vi "加速度曲線生成.vi"(0 "X Time":T1={"Time 1"=30.0, "Time 2"=60.0, "Time 3"=70.0, "Time 4"=80.0, "Time 5"=120.0, "Time 6"=180.0, "Time 7"=220.0, "Time 8"=300.0} {"Time 8" step=100.0; "Time 7" step=100.0; "Time 6" step=100.0; "Time 5" step=100.0; "Time 4" step=100.0; "Time 3" step=100.0; "Time 2" step=100.0; "Time 1" step=100.0}, 1 "Y Velocity":T2={"Speed 1"=70.0, "Speed 2"=-95.0, "Speed 3"=50.0, "Speed 4"=-50.0, "Speed 5"=60.0, "Speed 6"=-60.0, "Speed 7"=102.0, "Speed 8"=-80.0} {"Speed 8" step=100.0; "Speed 7" step=100.0; "Speed 6" step=100.0; "Speed 5" step=100.0; "Speed 4" step=100.0; "Speed 3" step=100.0; "Speed 2" step=100.0; "Speed 1" step=100.0}) -> (2 "Ideal Move":dbl[](array[numeric]), 3 "Ideal Acc":dbl[](array[numeric]), 4 "Voltage 1":dbl[](array[numeric]), 5 "Voltage 2":dbl[](array[numeric]), 6 "Voltage 3":dbl[](array[numeric]), 7 "Ideal Velocity":dbl[](array[numeric]))   [LabVIEW 2019]
uses:
  <vilib>/Analysis/NI_AALPro.lvlib
panel:
  out "Ideal Move Position Graph":cluster{"Speed":dbl[], "Position":dbl[]}(graph)
  out "Ideal S Graph":cluster{"Speed":dbl[], "Position":dbl[]}(graph)
  out "Ideal Velocity Graph":cluster{"Speed":dbl[], "Position":dbl[]}(graph)
  out "Ideal Axis 3 Voltage Position":cluster{dbl[], dbl[]}(graph)
  out "Ideal Axis 2 Voltage Position":cluster{dbl[], dbl[]}(graph)
  out "Ideal  Axis 1 Voltage Position":cluster{dbl[], dbl[]}(graph)
  out "Ideal Acceleration Graph":cluster{"Speed":dbl[], "Position":dbl[]}(graph)
  # "1mm/sec"
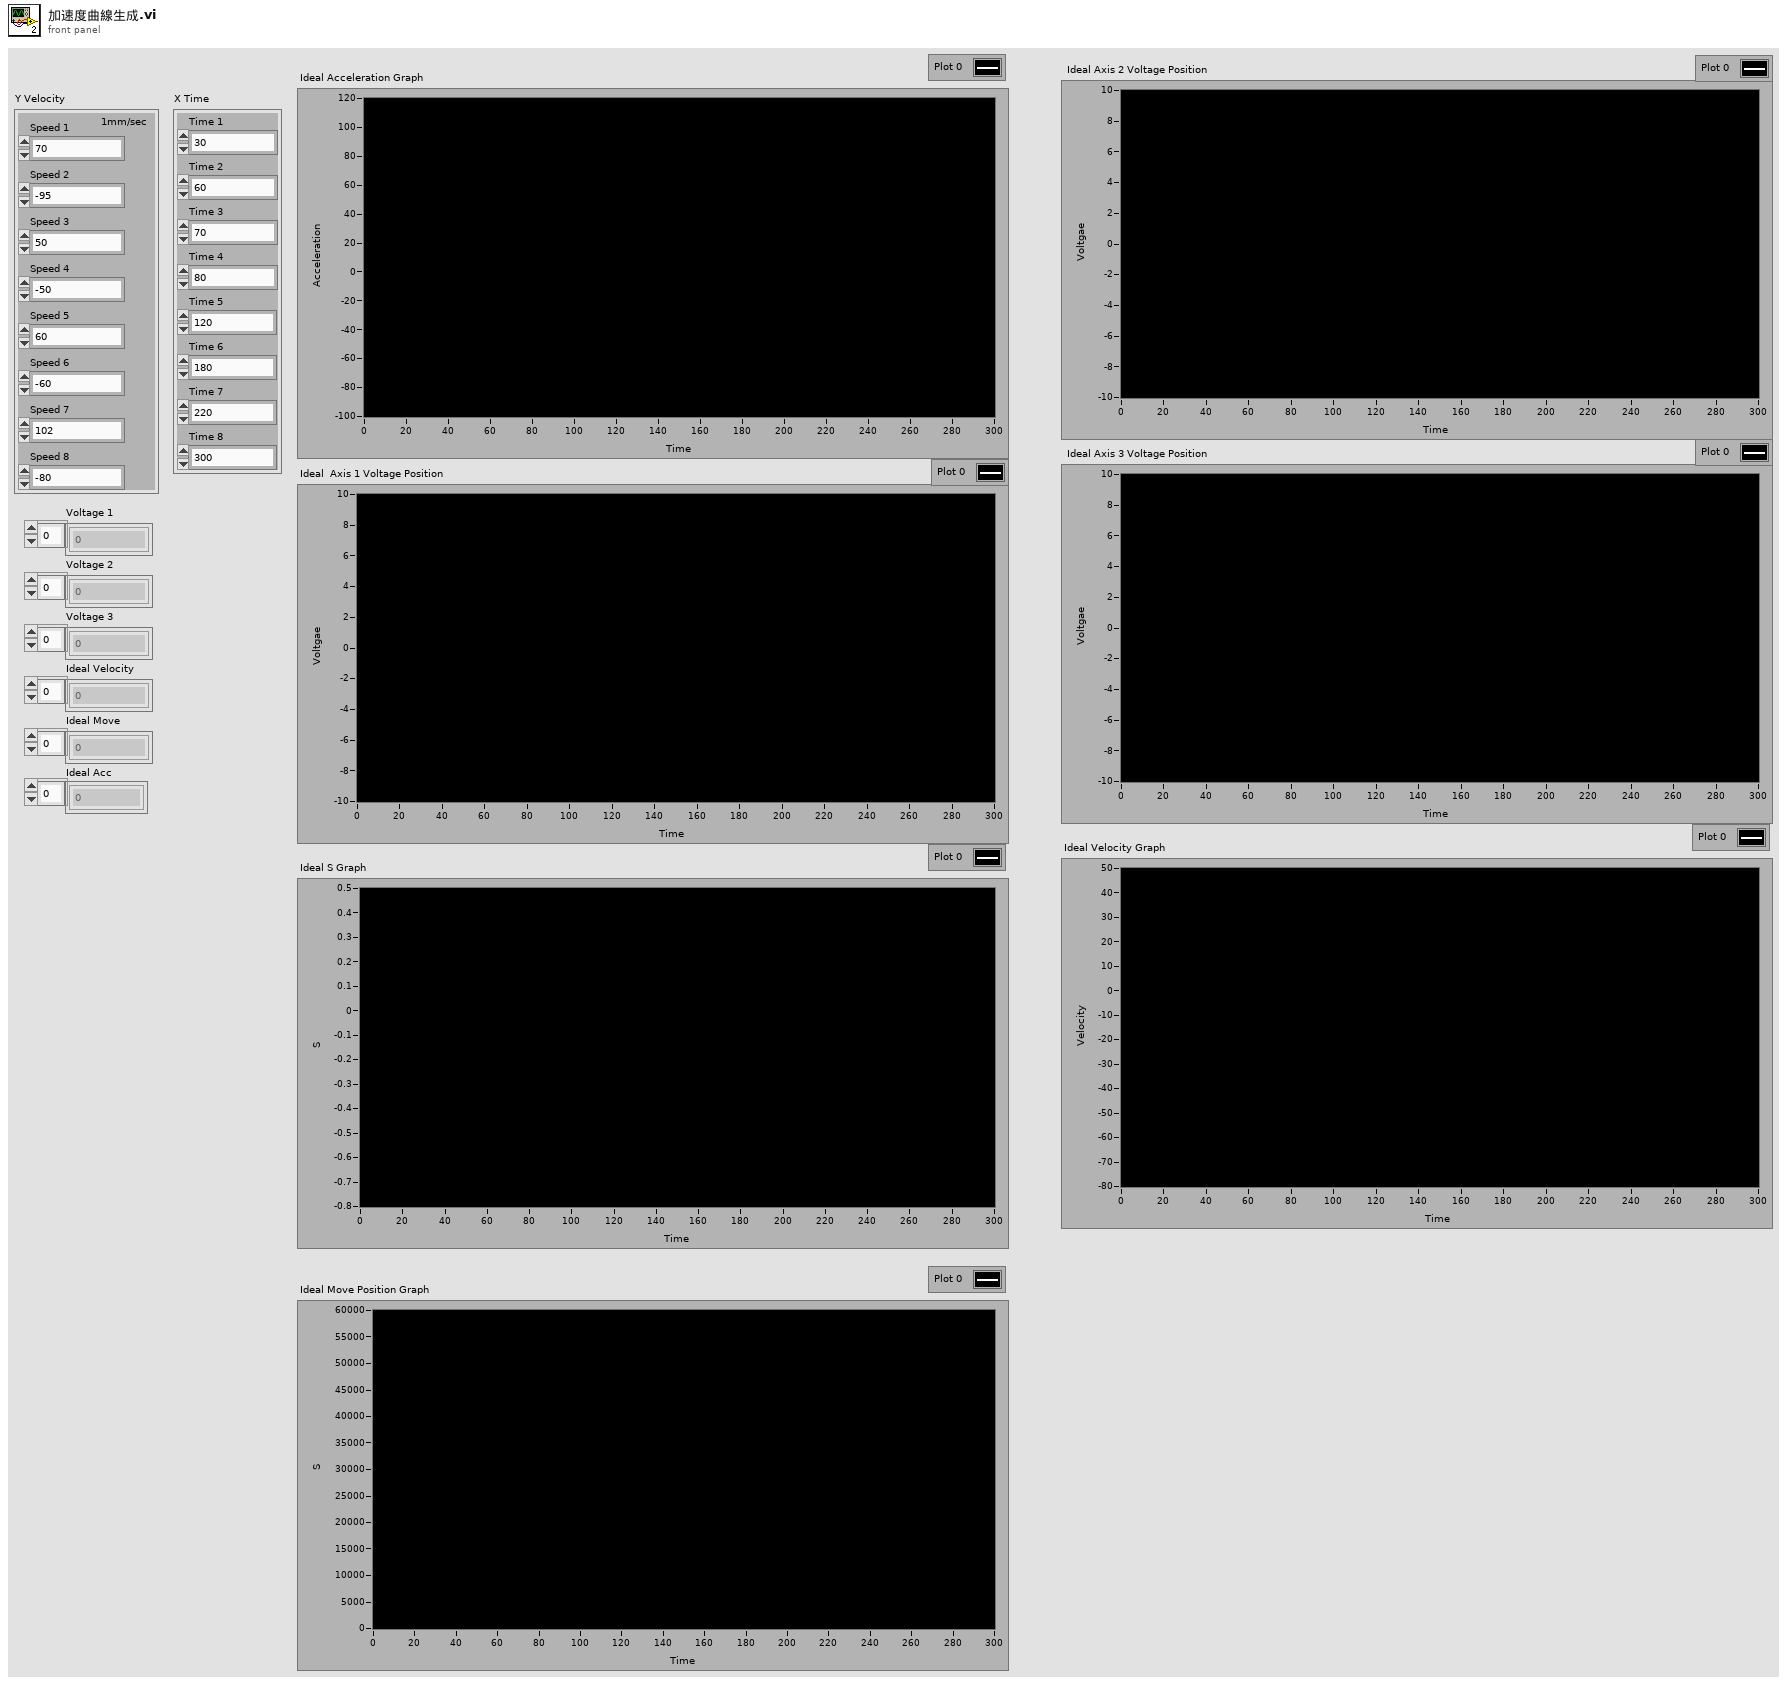
[diagram p1: front panel]
types:
  T1 = cluster{"Time 1":dbl, "Time 2":dbl, "Time 3":dbl, "Time 4":dbl, "Time 5":dbl, "Time 6":dbl, "Time 7":dbl, "Time 8":dbl}
  T2 = cluster{"Speed 1":dbl, "Speed 2":dbl, "Speed 3":dbl, "Speed 4":dbl, "Speed 5":dbl, "Speed 6":dbl, "Speed 7":dbl, "Speed 8":dbl}
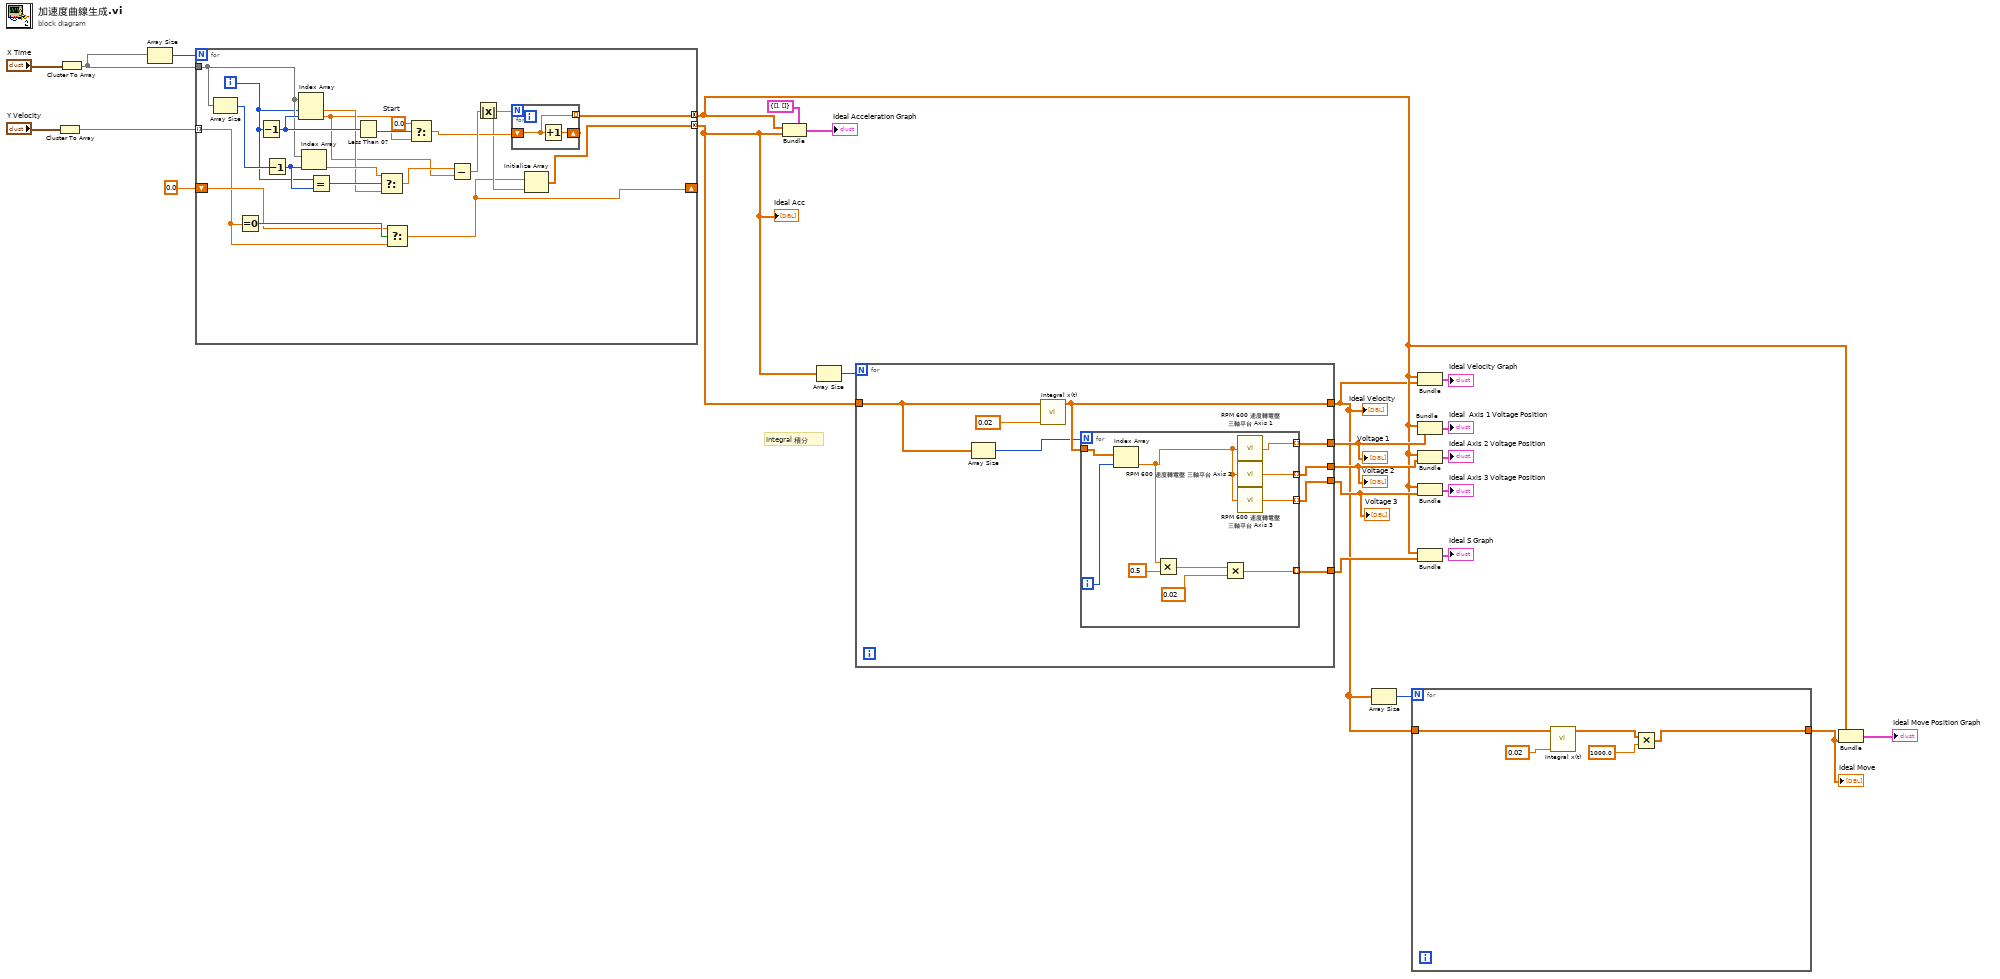
[diagram p0: block diagram]
diagram:
  # "Integral 積分"
  n1 = Cluster To Array(cluster="Y Velocity") -> (array=w20:dbl[])
  n2 = Cluster To Array(cluster="X Time") -> (array=w21:dbl[])
  n3 = Array Size(array=w21) -> (size(s)=w22:i32)
  n4 = for {
    N: w22 -> [_]
    tunnel: w21 -> [w42]
    tunnel: w20 -> [w29] mode=indexing
    shift-right: [w25] -> _
    shift-left: 0.0 -> [w30]
    tunnel: [w32] -> w4 mode=concatenating
    tunnel: [w28] -> w12 mode=concatenating
    i -> [w26]
    w43 = 0.0  # Start
    n5 = Array Size(array=w42) -> (size(s)=w39:i32)
    n6 = Equal To 0?(x=w29) -> (x = 0?=w31:bool)
    n7 = Decrement(x=w26) -> (x-1=w45:i32)
    n8 = Decrement(x=w39) -> (x-1=w40:i32)
    n9 = Index Array(array=w42, index #1=w26, index #2=w45) -> (element #1=w37:dbl, element #2=w33:dbl)
    n10 = Index Array(array=w42, index=w40) -> (element=w38:dbl)
    n11 = Equal?(x=w26, y=w40) -> (x = y?=w41:bool)
    n12 = Less Than 0?(x=w45) -> (x < 0?=w44:bool)
    n13 = Select(t=w38, s=w41, f=w37) -> (s? t:f=w34:dbl)
    n14 = Select(t=w30, s=w31, f=w29) -> (s? t:f=w25:dbl)
    n15 = Select(t=w43, s=w44, f=w33) -> (s? t:f=w35:dbl)
    n16 = Subtract(x=w34, y=w33) -> (x-y=w36:dbl)
    n17 = Absolute Value(x=w36) -> (abs(x)=w27:dbl)
    n18 = for {
      N: w27 -> [_]
      shift-right: [w47] -> _
      shift-left: w35 -> [w46]
      tunnel: [w46] -> w32 mode=indexing
      n19 = Increment(x=w46) -> (x+1=w47:dbl)
    }
    n20 = Initialize Array(w25, w27) -> (w28:dbl[])
  }
  "Ideal Acc" <- w12
  n21 = Bundle(cluster=cluster{"X Time":dbl[], "Y Velocity":dbl[]} {"X Time"=[], "Y Velocity"=[]}, "X Time"=w4, "Y Velocity"=w12) -> (→"Ideal Acceleration Graph":cluster{"X Time":dbl[], "Y Velocity":dbl[]})
  n22 = Array Size(array=w12) -> (size(s)=w11:i32)
  n23 = for {
    N: w11 -> [_]
    tunnel: [w54] -> w2
    tunnel: [w53] -> w6
    tunnel: [w51] -> w14
    tunnel: w12 -> [w48]
    tunnel: [w50] -> w8
    tunnel: [w49] -> w7
    n24 = Array Size(array=w48) -> (size(s)=w52:i32)
    n25 = call <vilib>:"Integral x(t).vi"("dt"=0.02, "X"=w48) -> ("Integral X"=w54:dbl[])  [unwired: 8 in, 1 out]
    n26 = for {
      N: w52 -> [_]
      tunnel: w54 -> [w63]
      tunnel: [w65] -> w53 mode=indexing
      tunnel: [w59] -> w51 mode=indexing
      tunnel: [w57] -> w50 mode=indexing
      tunnel: [w56] -> w49 mode=indexing
      i -> [w64]
      n27 = Index Array(array=w63, index=w64) -> (element=w58:dbl)
      n28 = Multiply(x=w58, y=0.5) -> (x*y=w61:dbl)
      n29 = Multiply(x=w61, y=0.02) -> (x*y=w59:dbl)
      n30 = call "RPM 600 速度轉電壓 三軸平台 Axis 1.vi"("Speed (1mm/s)"=w58) -> ("Voltage\nOutput"=w65:dbl)
      n31 = call "RPM 600 速度轉電壓 三軸平台 Axis 2.vi"("Speed (1mm/s)"=w58) -> ("Voltage\nOutput"=w57:dbl)
      n32 = call "RPM 600 速度轉電壓 三軸平台 Axis 3.vi"("Speed (1mm/s)"=w58) -> ("Voltage\nOutput"=w56:dbl)
    }
  }
  "Voltage 1" <- w6
  "Voltage 2" <- w8
  "Voltage 3" <- w7
  "Ideal Velocity" <- w2
  n33 = Array Size(array=w2) -> (size(s)=w5:i32)
  n34 = for {
    N: w5 -> [_]
    tunnel: w2 -> [w70]
    tunnel: [w66] -> w1
    n35 = call <vilib>:"Integral x(t).vi"("dt"=0.02 ("y"), "X"=w70) -> ("Integral X"=w68:dbl[])  [unwired: 8 in, 1 out]
    n36 = Multiply(x=w68, y=1000.0) -> (x*y=w66:dbl[])
  }
  "Ideal Move" <- w1
  n37 = Bundle(w4, "Integral X"=w2) -> (→"Ideal Velocity Graph":cluster{dbl[], "Integral X":dbl[]})  [unwired: 1 in]
  n38 = Bundle(w4, w6) -> (→"Ideal  Axis 1 Voltage Position":cluster{dbl[], dbl[]})  [unwired: 1 in]
  n39 = Bundle(w4, w8) -> (→"Ideal Axis 2 Voltage Position":cluster{dbl[], dbl[]})  [unwired: 1 in]
  n40 = Bundle(w4, w7) -> (→"Ideal Axis 3 Voltage Position":cluster{dbl[], dbl[]})  [unwired: 1 in]
  n41 = Bundle(w4, w14) -> (→"Ideal S Graph":cluster{dbl[], dbl[]})  [unwired: 1 in]
  n42 = Bundle(w4, w1) -> (→"Ideal Move Position Graph":cluster{dbl[], dbl[]})  [unwired: 1 in]
